vi "construct_response_send_I16_Waveform.vi"(0 "command in":T3=enum."configure_rf", 1 "Status":T2, 5 "generic_info":string, 7 "datatype":T1, 9 "I16 waveform in":i16[](array[numeric]), 11 "error in (no error) 2":errorcluster, 12 "source":string) -> (6 "Multipart message":string[](array[string]), 14 "parameters JSON":string, 15 "error out 2":errorcluster)   [LabVIEW 2019, in "mmW_commands.lvlib"]
uses:
  mmW_commands.lvlib
  TypeDefs/commands.ctl
  TypeDefs/response status.ctl
  typedefs/datatypes_.ctl
  typedefs/Response_paramaters.ctl
  <vilib>/addons/_JKI.lib/Serialization/JSON/JKI JSON Serialization.lvlib
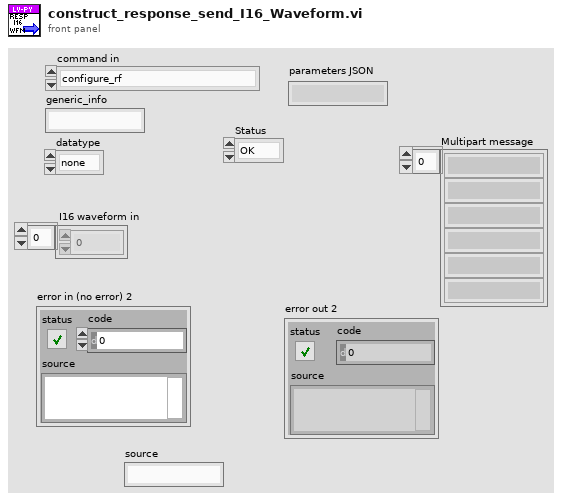
[diagram p1: front panel]
types:
  T1 = typedef "mmW_commands.lvlib/datatypes_.ctl" = enum16{"none", "string", "interleaved_I16", "interleaved_I32", "I16_array", "I32_array", "JSONstring"}
  T2 = typedef "mmW_commands.lvlib/response status.ctl" = enum16{"OK", "Error", "Warning", "Unknown"}
  T3 = typedef "mmW_commands.lvlib/commands.ctl" = enum16{"configure_fs", "configure_rf", "configure_trigger", "equalization_enable", "equalization_start", "lo_sync_enable", "equalization_stop", "get_instrument_status", "get_versions", "initialize_hw", "pop_rx", "set_log_level", "Shutdown", "start", "start_instrument_app", "stop", "trans", "transceive", "trigger_burst", "trigger_sync_enable", "Write TX", "resp_generic", "resp_waveform", "send_trigger", "fetch", "transceive2"}
  T4 = enum16{"big-endian, network order", "native, host order", "little-endian"}
  T5 = typedef "mmW_commands.lvlib/Response_paramaters.ctl" = cluster{"generic_info":string, "datatype":string, "source":string}
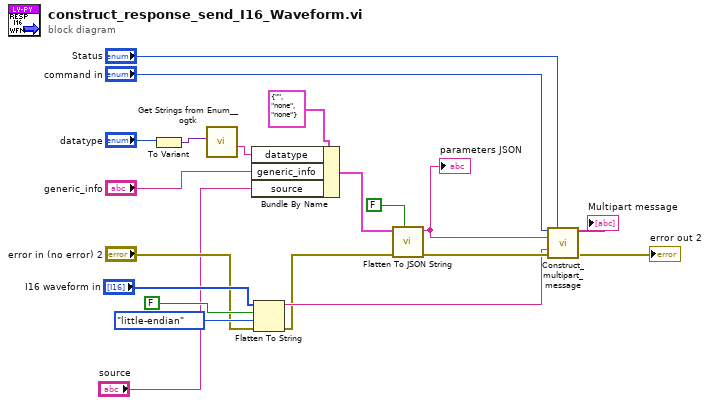
[diagram p0: block diagram]
diagram:
  n1 = To Variant(anything="datatype") -> (Variant=w9:variant)
  n2 = call <userlib>:"Get Strings from Enum__ogtk.vi"("Enum"=w9) -> ("String Value"=w8:string)  [unwired: 7 in, 3 out]
  n3 = Bundle By Name(cluster=T5 {"generic_info"="", "datatype"="none", "source"="none"} ("response data"), "datatype"=w8, "generic_info"="generic_info", "source"="source") -> (w19:T5)
  n4 = Flatten To String(anything="I16 waveform in", prepend array or string size? (T)=FALSE, byte order (0:big-endian, network order)=T4."little-endian", error in (no error)="error in (no error) 2") -> (data string=w3:string, error out=w2:errorcluster)  [unwired: 1 out]
  n5 = call <vilib>:"Flatten To JSON String.vi"("Multiline (T)"=FALSE, "error in (no error)"=w2, "Variant"=w19) -> ("error out"=w15:errorcluster, "JSON String"=w16:string)  [unwired: 7 in]
  "parameters JSON" <- w16
  n6 = call "Construct_multipart_message.vi"("command"="command in", "Status"="Status", "parameters (JSON)"=w16, "data in"=w3, "error in (no error)"=w15) -> ("Multipart message"=→"Multipart message":string[], "error out"=→"error out 2":errorcluster)  [unwired: 7 in, 2 out]
